vi "Edgertronic-get_storage_dir.vi"(3 "error in (no error)":errorcluster, 5 "URL":string="192.168.1.101") -> (0 "error out":errorcluster={"status"=FALSE, "code"=66, "source"="TCP Read in Edgertronic-GET_cmd.vi->Edgertronic-get_storage_dir.vi"}, 1 "Storage Dir:":T1={"Storage Dir"="/mnt/sdcard", "Connection Information:"="HTTP/1.0 200 OK\r\nContent-Type: text/html; charset=utf-8\r\nContent-Length: 13\r\nConnection: close\r\nDate: Tue, 14 Jun 2016 12:17:05 GMT\r\nServer: lighttpd/1.4.11 (edgertonic slow motion camera)"})   [LabVIEW 2015]
doc: "This VI returns the mount point of the active storage device."
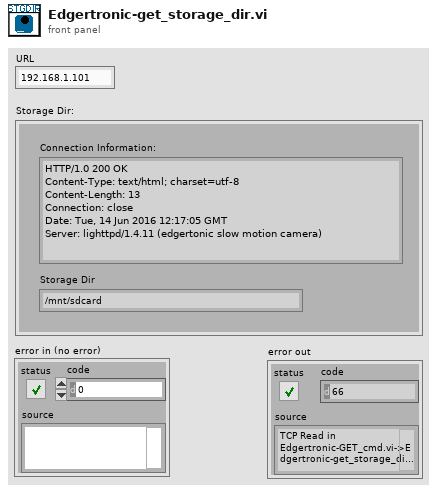
[diagram p1: front panel]
types:
  T1 = cluster{"Storage Dir":string, "Connection Information:":string}
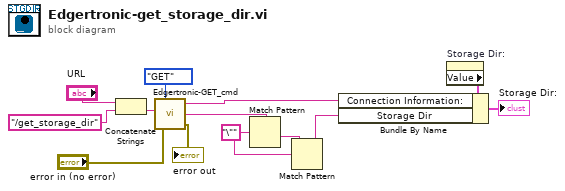
[diagram p0: block diagram]
diagram:
  w7 = "\"" ("regular expression")
  n1 = Concatenate Strings("URL", "/get_storage_dir" ("GET Cmd")) -> (w2:string)
  n2 = call "Edgertronic-GET_cmd.vi"("error in (no error)"="error in (no error)", "URL"=w2, "Type"=enum16{"GET", "POST"}."GET") -> ("error out"=→"error out":errorcluster, "data"=w9:string, "Connection Info"=w10:string)  [unwired: 1 in]
  n3 = Match Pattern(string=w9, regular expression=w7) -> (after substring=w8:string)  [unwired: 1 in, 3 out]
  n4 = Match Pattern(string=w8, regular expression=w7) -> (before substring=w6:string)  [unwired: 1 in, 3 out]
  n5 = property on="Storage Dir:" class="Clust (strict)"() -> ("Value"=w11:T1)  [unwired: 2 in, 2 out]
  n6 = Bundle By Name(cluster=w11, "Connection Information:"=w10, "Storage Dir"=w6) -> (→"Storage Dir:":T1)
